vi "GetIniInfo.vi"(8 "error in (no error)":errorcluster, 10 "PathToIni":path, 11 "BasePath":path) -> (0 "error out":errorcluster, 2 "clConfig":T1={"F0"=60, "SettlingTime"=7.0, "AnalysisCycles"=20.0, "SampleRate"=4800.0, "NumChannels"=6, "TsOffset"=enum."start"}, 3 "PathToClass":path)   [LabVIEW 2014, in "AnalysisPlugins.lvlib" / "AnalysisPluginsBase.lvclass"]
uses:
  AnalysisPluginsBase.lvclass
  Typedefs/clConfig.ctl
  <userlib>/NIST/BaseClasses/Object_class/BaseObject.lvclass
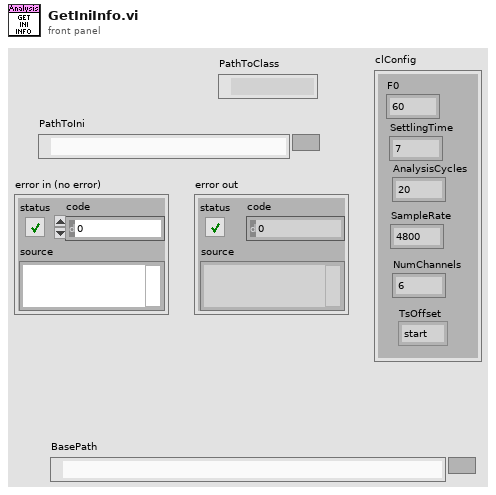
[diagram p1: front panel]
types:
  T1 = typedef "AnalysisPlugins.lvlib/AnalysisPluginsBase.lvclass/clConfig.ctl" = cluster{"F0":u32, "SettlingTime":dbl, "AnalysisCycles":dbl, "SampleRate":dbl, "NumChannels":u32, "TsOffset":enum16{"start", "middle", "end"}}
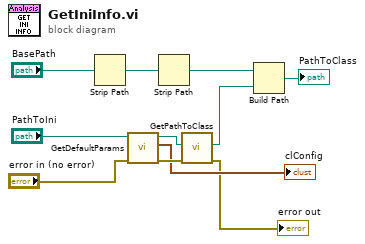
[diagram p0: block diagram]
diagram:
  n1 = Strip Path(path="BasePath") -> (stripped path=w2:path)  [unwired: 1 out]
  n2 = call "GetDefaultParams.vi"("error in (no error)"="error in (no error)", "PathToIni"="PathToIni") -> ("error out"=w8:errorcluster, "clConfig"=→"clConfig":T1, "PathToClass"=w6:path)  [unwired: 7 in]
  n3 = Strip Path(path=w2) -> (stripped path=w1:path)  [unwired: 1 out]
  n4 = call <userlib>:"GetPathToClass.vi"("error in (no error)"=w8, "configuration file path"=w6) -> ("error IO"=→"error out":errorcluster, "PathToClass"=w5:path)  [unwired: 8 in]
  n5 = Build Path(base path=w1, name or relative path=w5) -> (appended path=→"PathToClass":path)
